vi "220121_xiang_calibration data analysis.vi"() -> ()   [LabVIEW 2020]
uses:
  OldDAQtask/CylinderCalibration/XYZE_power_spectra.ctl
  OldDAQtask/CylinderCalibration/single_power_spectrum.ctl
  OldDAQtask/CylinderCalibration/XYZ scan data.ctl
  OldDAQtask/CylinderCalibration/fast winding result.ctl
  <vilib>/Analysis/baseanly.llb/Mean (DBL).vi
  <vilib>/Utility/file.llb/Write To Spreadsheet File (DBL).vi
  Initialization/FileManagement/FileManagement.lvlib
  OldDAQtask/HeightFinder/HeightFinder.lvlib
  <vilib>/Analysis/NI_AALPro.lvlib
  <vilib>/Analysis/NI_AALBase.lvlib
  OldDAQtask/CylinderCalibration/CylinderCalibration.lvlib
panel:
  out "Array 2":dbl[][](array[numeric])
  out "Array":dbl[][](array[numeric])
  out "error out":errorcluster
  out "pb1":dbl(slide)=1.0 scale=0.0..1.0
  in  "kT_pNnm":dbl=4.09
  in  "stop":bool
  in  "cylinder list":i32[](listbox)
  in  "root path":path=path "Y:/Setup4/Xiaomeng/220107_Xiaomeng_q30 calibration"
  in  "Tab Control":T1(tab)=enum."averaged result"
  out "ellipticity vs angle":cluster{dbl[], dbl[]}[](graph)
  out "max ellipticity vs power":cluster{dbl[], dbl[]}[](graph)
  out "x variance vs angle":cluster{dbl[], dbl[]}[](graph)
  out "y variance vs angle":cluster{dbl[], dbl[]}[](graph)
  out "z variance vs angle":cluster{dbl[], dbl[]}[](graph)
  out "ellipticity fitting":cluster{dbl[], dbl[]}[](graph)
  out "z signal fitting":cluster{dbl[], dbl[]}[](graph)
  out "x signal fitting":cluster{dbl[], dbl[]}[](graph)
  out "y signal fitting":cluster{dbl[], dbl[]}[](graph)
  out "var ellipticity vs power":cluster{dbl[], dbl[]}[](graph)
  out "var x signal vs power":cluster{dbl[], dbl[]}[](graph)
  out "var y signal vs power":cluster{dbl[], dbl[]}[](graph)
  out "var z signal vs power":cluster{dbl[], dbl[]}[](graph)
  out "x DoG":cluster{dbl[], dbl[]}[](graph)
  out "y DoG":cluster{dbl[], dbl[]}[](graph)
  out "z DoG":cluster{dbl[], dbl[]}[](graph)
  out "Height finder data":cluster{dbl[], "Best Polynomial Fit":dbl[]}[](graph)
  out "original calibration file":string="[Trap and cylinder calibration]\nKz, pN/nm/W=0.349554\nKx, pN/nm/W=0.376339\nKy, pN/nm/W=0.248999\nSz, 1/nm=0.000578\nSx, 1/nm=0.000761\nSy, 1/nm=0.000667\nKang, pNnm/rad/W=17149.300335\nMax ellipticity, 1=0.032157\nFocal shift=0.790000\nZsignalHeightDependence, 1/nm=0\n[Piezo AO calibration and settings]\nVx/Px(V/nm)=0.000667\nVy/Py(V/nm)=0.000667\nVz/Pz(V/nm)=0.002000\nMax Px (nm)=30000.000000\nMax Py (nm)=30000.000000\nMax Pz (nm)=10000.000000\nMin Px (nm)=0.000000\nMin Py (nm)=0.000000\nMin Pz (nm)=0.000000\nVx0 (V)=-10.000000\nVy0 (V)=-10.000000\nVz0 (V)=-10.000000\nAI2p=1.101000E+4\\095.746000E+3\\093.323000E+0\\0D\\0A1.016000E+4\\095.766000E+3\\093.739000E+0\\0D\\0A6.154000E+3\\095.319000E+3\\091.621000E+1\\0D\\0A\n[matrix Mp2s (3X3)]\na11=1.000000\na12=0.000000\na13=0.000000\na21=0.000000\na22=1.000000\na23=0.000000\na31=0.000000\na32=0.000000\na33=1.000000\n[DAQ settings]\nAIBufferSize=100000\nDAQ ScanRate=10000\nPoints to average=20\nSamping rate=500\n[PS detector signal to laser power (W) conversion matrix (2X2)]\na11=0.0152532\na12=-0.00000458129\na21=-0.0000113255\na22=0.0139626\n[Z bead vs Z signal polynomial coefficients (nm)]\na0=0.000000\na1=1773.000000\na2=0.000000\na3=0.000000\na4=0.000000\na5=0.000000\n[Z bead look up table]\n(Z signal, Z bead)=-1.000000E+2\\09-4.925198E+2\\0D\\0A-2.068564E-1\\09-4.740681E+2\\0D\\0A-2.031962E-1\\09-4.583933E+2\\0D\\0A-1.995359E-1\\09-4.445056E+2\\0D\\0A-1.958757E-1\\09-4.317229E+2\\0D\\0A-1.922155E-1\\09-4.195962E+2\\0D\\0A-1.885553E-1\\09-4.078497E+2\\0D\\0A-1.848951E-1\\09-3.963318E+2\\0D\\0A-1.812349E-1\\09-3.849767E+2\\0D\\0A-1.775747E-1\\09-3.737744E+2\\0D\\0A-1.739145E-1\\09-3.627475E+2\\0D\\0A-1.702543E-1\\09-3.519346E+2\\0D\\0A-1.665941E-1\\09-3.413777E+2\\0D\\0A-1.629339E-1\\09-3.311145E+2\\0D\\0A-1.592737E-1\\09-3.211728E+2\\0D\\0A-1.556135E-1\\09-3.115682E+2\\0D\\0A-1.519532E-1\\09-3.023034E+2\\0D\\0A-1.482930E-1\\09-2.933685E+2\\0D\\0A-1.446328E-1\\09-2.847427E+2\\0D\\0A-1.409726E-1\\09-2.763963E+2\\0D\\0A-1.373124E-1\\09-2.682934E+2\\0D\\0A-1.336522E-1\\09-2.603938E+2\\0D\\0A-1.299920E-1\\09-2.526561E+2\\0D\\0A-1.263318E-1\\09-2.450395E+2\\0D\\0A-1.226716E-1\\09-2.375059E+2\\0D\\0A-1.190114E-1\\09-2.300210E+2\\0D\\0A-1.153512E-1\\09-2.225562E+2\\0D\\0A-1.116910E-1\\09-2.150888E+2\\0D\\0A-1.080307E-1\\09-2.076026E+2\\0D\\0A-1.043705E-1\\09-2.000879E+2\\0D\\0A-1.007103E-1\\09-1.925414E+2\\0D\\0A-9.705012E-2\\09-1.849654E+2\\0D\\0A-9.338991E-2\\09-1.773671E+2\\0D\\0A-8.972970E-2\\09-1.697580E+2\\0D\\0A-8.606949E-2\\09-1.621523E+2\\0D\\0A-8.240929E-2\\09-1.545665E+2\\0D\\0A-7.874908E-2\\09-1.470176E+2\\0D\\0A-7.508887E-2\\09-1.395227E+2\\0D\\0A-7.142866E-2\\09-1.320976E+2\\0D\\0A-6.776845E-2\\09-1.247560E+2\\0D\\0A-6.410824E-2\\09-1.175090E+2\\0D\\0A-6.044804E-2\\09-1.103642E+2\\0D\\0A-5.678783E-2\\09-1.033255E+2\\0D\\0A-5.312762E-2\\09-9.639297E+1\\0D\\0A-4.946741E-2\\09-8.956269E+1\\0D\\0A-4.580720E-2\\09-8.282687E+1\\0D\\0A-4.214700E-2\\09-7.617425E+1\\0D\\0A-3.848679E-2\\09-6.959053E+1\\0D\\0A-3.482658E-2\\09-6.305893E+1\\0D\\0A-3.116637E-2\\09-5.656087E+1\\0D\\0A-2.750616E-2\\09-5.007675E+1\\0D\\0A-2.384595E-2\\09-4.358670E+1\\0D\\0A-2.018575E-2\\09-3.707141E+1\\0D\\0A-1.652554E-2\\09-3.051286E+1\\0D\\0A-1.286533E-2\\09-2.389508E+1\\0D\\0A-9.205121E-3\\09-1.720474E+1\\0D\\0A-5.544913E-3\\09-1.043171E+1\\0D\\0A-1.884705E-3\\09-3.569408E+0\\0D\\0A1.775503E-3\\093.384973E+0\\0D\\0A5.435712E-3\\091.043038E+1\\0D\\0A9.095920E-3\\091.756204E+1\\0D\\0A1.275613E-2\\092.477176E+1\\0D\\0A1.641634E-2\\093.204839E+1\\0D\\0A2.007654E-2\\093.937846E+1\\0D\\0A2.373675E-2\\094.674700E+1\\0D\\0A2.739696E-2\\095.413840E+1\\0D\\0A3.105717E-2\\096.153747E+1\\0D\\0A3.471738E-2\\096.893042E+1\\0D\\0A3.837759E-2\\097.630600E+1\\0D\\0A4.203779E-2\\098.365648E+1\\0D\\0A4.569800E-2\\099.097859E+1\\0D\\0A4.935821E-2\\099.827434E+1\\0D\\0A5.301842E-2\\091.055516E+2\\0D\\0A5.667863E-2\\091.128245E+2\\0D\\0A6.033884E-2\\091.201134E+2\\0D\\0A6.399904E-2\\091.274448E+2\\0D\\0A6.765925E-2\\091.348504E+2\\0D\\0A7.131946E-2\\091.423665E+2\\0D\\0A7.497967E-2\\091.500322E+2\\0D\\0A7.863988E-2\\091.578880E+2\\0D\\0A8.230008E-2\\091.659733E+2\\0D\\0A8.596029E-2\\091.743245E+2\\0D\\0A8.962050E-2\\091.829723E+2\\0D\\0A9.328071E-2\\091.919395E+2\\0D\\0A9.694092E-2\\092.012384E+2\\0D\\0A1.006011E-1\\092.108698E+2\\0D\\0A1.042613E-1\\092.208213E+2\\0D\\0A1.079215E-1\\092.310681E+2\\0D\\0A1.115818E-1\\092.415750E+2\\0D\\0A1.152420E-1\\092.523003E+2\\0D\\0A1.189022E-1\\092.632031E+2\\0D\\0A1.225624E-1\\092.742540E+2\\0D\\0A1.262226E-1\\092.854502E+2\\0D\\0A1.298828E-1\\092.968364E+2\\0D\\0A1.335430E-1\\093.085323E+2\\0D\\0A1.372032E-1\\093.207678E+2\\0D\\0A1.408634E-1\\093.339281E+2\\0D\\0A1.445236E-1\\093.486096E+2\\0D\\0A1.481838E-1\\093.656889E+2\\0D\\0A1.000000E+2\\093.864067E+2\\0D\\0A\n[Comment from Q30 Calibration] 10 mM Tris-HCl, pH = 8; 40 mM MgCl2; 50 mM NaCl; 0.2 mg/mL beta-casein\n1/14/2021 11:33 AM"
  out "Updated calibration file":string
  out "Updated calibration file location":path
  out "SD of force sensitivity, pN/W":dbl=12.607172653733816
  out "SEM of force sensitivity, pN/W":dbl=3.151793163433454
  out "force sensitivity, pN/W":dbl=492.26794237481425
  out "SD of torque sensitivity, pNnm/W":dbl=244140.75454887396
  out "SEM of torque sensitivity, pNnm/W":dbl=61035.18863721849
  out "torque sensitivity, pNnm/W":dbl=308105.85527126427
  out "SD of z stiffness, pN/nm/W":dbl=0.006440898726546468
  out "SD of z sensitivity, 1/nm":dbl=5.569909992065383e-06
  out "SD of angular stifness, pNnm/rad/W":dbl=320.0752807876521
  out "SD of angular sensitivity, 1/rad":dbl=0.00035066082703313163
  out "z force sensitivity":T2(graph)={"final result"=[1.0, 2.0, 3.0, 4.0, 6.0, 7.0], "final result"=[498.4071904780335, 474.8213008025603, 504.1808261472068, 495.5040400134854, 478.2463154671384, 502.4479813404608]}
  out "Torque sensitivity":T2(graph)={"final result"=[1.0, 2.0, 3.0, 4.0, 6.0, 7.0], "final result"=[73.67021354183011, -8913.301705379306, 498179.1915137824, 417955.8385778271, 442478.0259262357, 498861.70710157783]}
  out "SEM of z stiffness, pN/nm/W":dbl=0.001610224681636617
  out "z stiffness, pN/nm/W":dbl=0.16169724642273595
  out "SEM of z sensitivity, 1/nm":dbl=1.3924774980163457e-06
  out "z sensitivity, 1/nm":dbl=0.00032838353115096313
  out "SEM of angular stifness, pNnm/rad/W":dbl=80.01882019691303
  out "angular stiffness, pNnm/rad/W":dbl=375.5197105345397
  out "SEM of angular sensitivity, 1/rad":dbl=8.766520675828291e-05
  out "angular sensitivity, 1/rad":dbl=0.0013622152574613259
  out "final result":dbl[][](array[numeric])=[[1.0, 2.0, 3.0, 4.0, 6.0, 7.0], [nan, nan, nan, nan, nan, nan], [0.13279234841776086, -13.36709953944761, 674.8537139952265, 372.11897404124767, 711.6919827860539, 507.68789957574], [0.0018025242772285583, 0.001499679914501309, 0.0013546405098627172, 0.0008903308428647679, 0.0016084233364951283, 0.001017692663815475], [73.67021354183011, -8913.301705379306, 498179.1915137824, 417955.8385778271, 442478.0259262357, 498861.70710157783], [0.16579227343626485, 0.1513303954658166, 0.16883942461520451, 0.16284381884534085, 0.15689235695361436, 0.16448520922017446], [0.00033264422464942726, 0.00031871020784036524, 0.0003348787098974448, 0.00032864276715263306, 0.0003280576386675683, 0.00032736763869834043], [498.4071904780335, 474.8213008025603, 504.1808261472068, 495.5040400134854, 478.2463154671384, 502.4479813404608], [0.6695465077566299, 0.9654608095555708, 1.1766726492381052, 1.2199767576089258, 1.1806760501666687, 0.7481024842794938], [0.0006195077361526612, 0.0007552886971877524, 0.0008161495017131666, 0.0008342978728837841, 0.0008284250298047227, 0.0006508474644543304], [1080.771826861639, 1278.267254826366, 1441.7366509054655, 1462.279597324187, 1425.205670626561, 1149.428284101409], [0.7539490293969152, 0.9600841428867122, 1.1413404013712398, 1.013487614262731, 1.027256013548298, 0.8640080844160597], [0.0005940302228699274, 0.0006707172355041432, 0.0007217134695992056, 0.0007028215814044456, 0.000725406642994016, 0.0006430202724935601], [1269.2098825449907, 1431.4290614062822, 1581.4314813953365, 1442.0268828932126, 1416.1105684233055, 1343.6716093965963], [0.19148344824695612, 0.21192606642906414, 0.19576149623991493, 0.19479979524743082, 0.19336718080202564, 0.19576422973039367], [0.12166886063179862, 0.12359792221219097, 0.12170898606033095, 0.12101974277514069, 0.11972394587250185, 0.12216359051715364]]
  out "z sensitivity":T2(graph)={"final result"=[1.0, 2.0, 3.0, 4.0, 6.0, 7.0], "final result"=[0.00033264422464942726, 0.00031871020784036524, 0.0003348787098974448, 0.00032864276715263306, 0.0003280576386675683, 0.00032736763869834043]}
  out "Angular sensitivity":T2(graph)={"final result"=[1.0, 2.0, 3.0, 4.0, 6.0, 7.0], "final result"=[0.0018025242772285583, 0.001499679914501309, 0.0013546405098627172, 0.0008903308428647679, 0.0016084233364951283, 0.001017692663815475]}
  out "max z force, pN/W":dbl=97.02091670635467
  out "SEM of max z force, pN/W":dbl=0.7160625967795665
  out "SD of max z force, pN/W":dbl=2.864250387118266
  out "Maximum torque":T2(graph)={"final result"=[1.0, 2.0, 3.0, 4.0, 6.0, 7.0], "final result"=[0.06639617420888043, -6.683549769723805, 337.42685699761324, 186.05948702062383, 355.84599139302696, 253.84394978787]}
  out "Maximum z force":T2(graph)={"final result"=[1.0, 2.0, 3.0, 4.0, 6.0, 7.0], "final result"=[95.43672746381132, 100.62701053581804, 98.69919290205362, 96.52408553890173, 92.47714175083674, 98.36134204670653]}
  out "Angular stiffness":T2(graph)={"final result"=[1.0, 2.0, 3.0, 4.0, 6.0, 7.0], "final result"=[0.13279234841776086, -13.36709953944761, 674.8537139952265, 372.11897404124767, 711.6919827860539, 507.68789957574]}
  out "z stiffness":T2(graph)={"final result"=[1.0, 2.0, 3.0, 4.0, 6.0, 7.0], "final result"=[0.16579227343626485, 0.1513303954658166, 0.16883942461520451, 0.16284381884534085, 0.15689235695361436, 0.16448520922017446]}
  out "CV of max z force":dbl=0.029521988498493166
  out "CV of angular sensitivity":dbl=0.2574195415243226
  out "CV of angular stifness":dbl=0.8523528108072828
  out "CV of z sensitivity":dbl=0.016961599665315758
  out "CV of z stiffness":dbl=0.03983307612862866
  out "CV of torque sensitivity":dbl=0.7923924533466792
  out "CV of force sensitivity":dbl=0.02561038728809742
  out "mean":dbl[](array[numeric])=[3.8333333333333335, nan, 375.5197105345397, 0.0013622152574613259, 308105.85527126427, 0.16169724642273595, 0.00032838353115096313, 492.26794237481425, 0.9934058764342324, 0.0007507527170327362, 1306.2815474409379, 0.960020880980326, 0.0006762849041442163, 1413.9799143432874, 0.1971837027826309, 0.12164717467818613]
  out "SD":dbl[](array[numeric])=[2.3166067138525404, nan, 320.0752807876521, 0.00035066082703313163, 244140.75454887396, 0.006440898726546468, 5.569909992065383e-06, 12.607172653733816, 0.2390944431916935, 9.435719400130207e-05, 163.137245645585, 0.13560242786564763, 5.115518013146681e-05, 104.91643534205578, 0.007404277385621852, 0.0012781918494249795]
  out "x stiffness":T2(graph)={"final result"=[1.0, 2.0, 3.0, 4.0, 6.0, 7.0], "final result"=[0.6695465077566299, 0.9654608095555708, 1.1766726492381052, 1.2199767576089258, 1.1806760501666687, 0.7481024842794938]}
  out "Maximum x force":T2(graph)={"final result"=[1.0, 2.0, 3.0, 4.0, 6.0, 7.0], "final result"=[60.64063499615816, 58.68692620128618, 61.36333714143654, 59.96577146647502, 57.25753598671112, 61.38084944864651]}
  out "x sensitivity":T2(graph)={"final result"=[1.0, 2.0, 3.0, 4.0, 6.0, 7.0], "final result"=[0.0006195077361526612, 0.0007552886971877524, 0.0008161495017131666, 0.0008342978728837841, 0.0008284250298047227, 0.0006508474644543304]}
  out "x force sensitivity":T2(graph)={"final result"=[1.0, 2.0, 3.0, 4.0, 6.0, 7.0], "final result"=[1080.771826861639, 1278.267254826366, 1441.7366509054655, 1462.279597324187, 1425.205670626561, 1149.428284101409]}
  out "max x force, pN/W":dbl=59.882509206785585
  out "SD of max x force, pN/W":dbl=1.6333686233039957
  out "SEM of max x force, pN/W":dbl=0.4083421558259989
  out "CV of max x force":dbl=0.027276222137981327
  out "x stiffness, pN/nm/W":dbl=0.9934058764342324
  out "SEM of x stiffness, pN/nm/W":dbl=0.05977361079792338
  out "SD of x stiffness, pN/nm/W":dbl=0.2390944431916935
  out "CV of x stiffness":dbl=0.24068152692020295
  out "z sensitivity, 1/nm 2":dbl=0.0007507527170327362
  out "SEM of z sensitivity, 1/nm 2":dbl=2.358929850032552e-05
  out "SD of z sensitivity, 1/nm 2":dbl=9.435719400130207e-05
  out "CV of z sensitivity 2":dbl=0.1256834532337599
  out "Comment":string
  out "Name":string
  in  "fast winding results":T3[](array[typedef]) {"Laser power before obj[W]" format="%.4f"; "relative fluctuation (fluctuation/mean)" format="%#_6e"; "mean e amplitude" format="%#_6e"}
  in  "stifness results":T4[][](array[typedef]) {"result of y signal"."var" format="%.3e"; "result of y signal"."sigma^2" format="%.3e"; "result of x signal"."var" format="%.3e"; "result of x signal"."sigma^2" format="%.3e"; "result of z signal"."var" format="%.3e"; "result of z signal"."sigma^2" format="%.3e"; "result of ellipticity"."var" format="%.3e"; "result of ellipticity"."sigma^2" format="%.3e"; "general info"."Time/Date" format="%<%.3X, %x>T"}
  in  "XYZ scan result":T6 {"y_signal vs trap height slope around eq position, 1/nm" format="%#.6g"; "x_signal vs trap height slope around eq position, 1/nm" format="%#.6g"; "Zsig baseline" format="%#.6g"; "Xsig baseline" format="%#.6g"; "Ysig baseline" format="%#.6g"; "z_signal vs trap height slope around eq position, 1/nm" format="%#.6g"}
  out "distance between trap center and z DoG center":dbl[](array[numeric])
  out "only use slopes":dbl[][](array[numeric]) format="%_3e"
  out "intercepts that will be ignored":dbl[][](array[numeric]) format="%_3e"
  # "column name:\n\n0: Cylinder No.\n1: Good? (=1)\n2: K_theta\n3: S_theta\n4: K_e\n5: K_z\n6: S_z\n7: K_zsig\n8: K_x\n9: S_x\n10: K_xsig\n11: K_y\n12: S_y\n13: K_ysig\n14: Max z signal\n15: Max x signal"
  # "Rows:\n\n0: Cylinder No.\n1: \n2: K_theta\n3: S_theta\n4: K_e\n5: K_z\n6: S_z\n7: K_zsig\n8: K_x\n9: S_x\n10: K_xsig\n11: K_y\n12: S_y\n13: K_ysig\n14: Max z signal\n15: Max x signal"
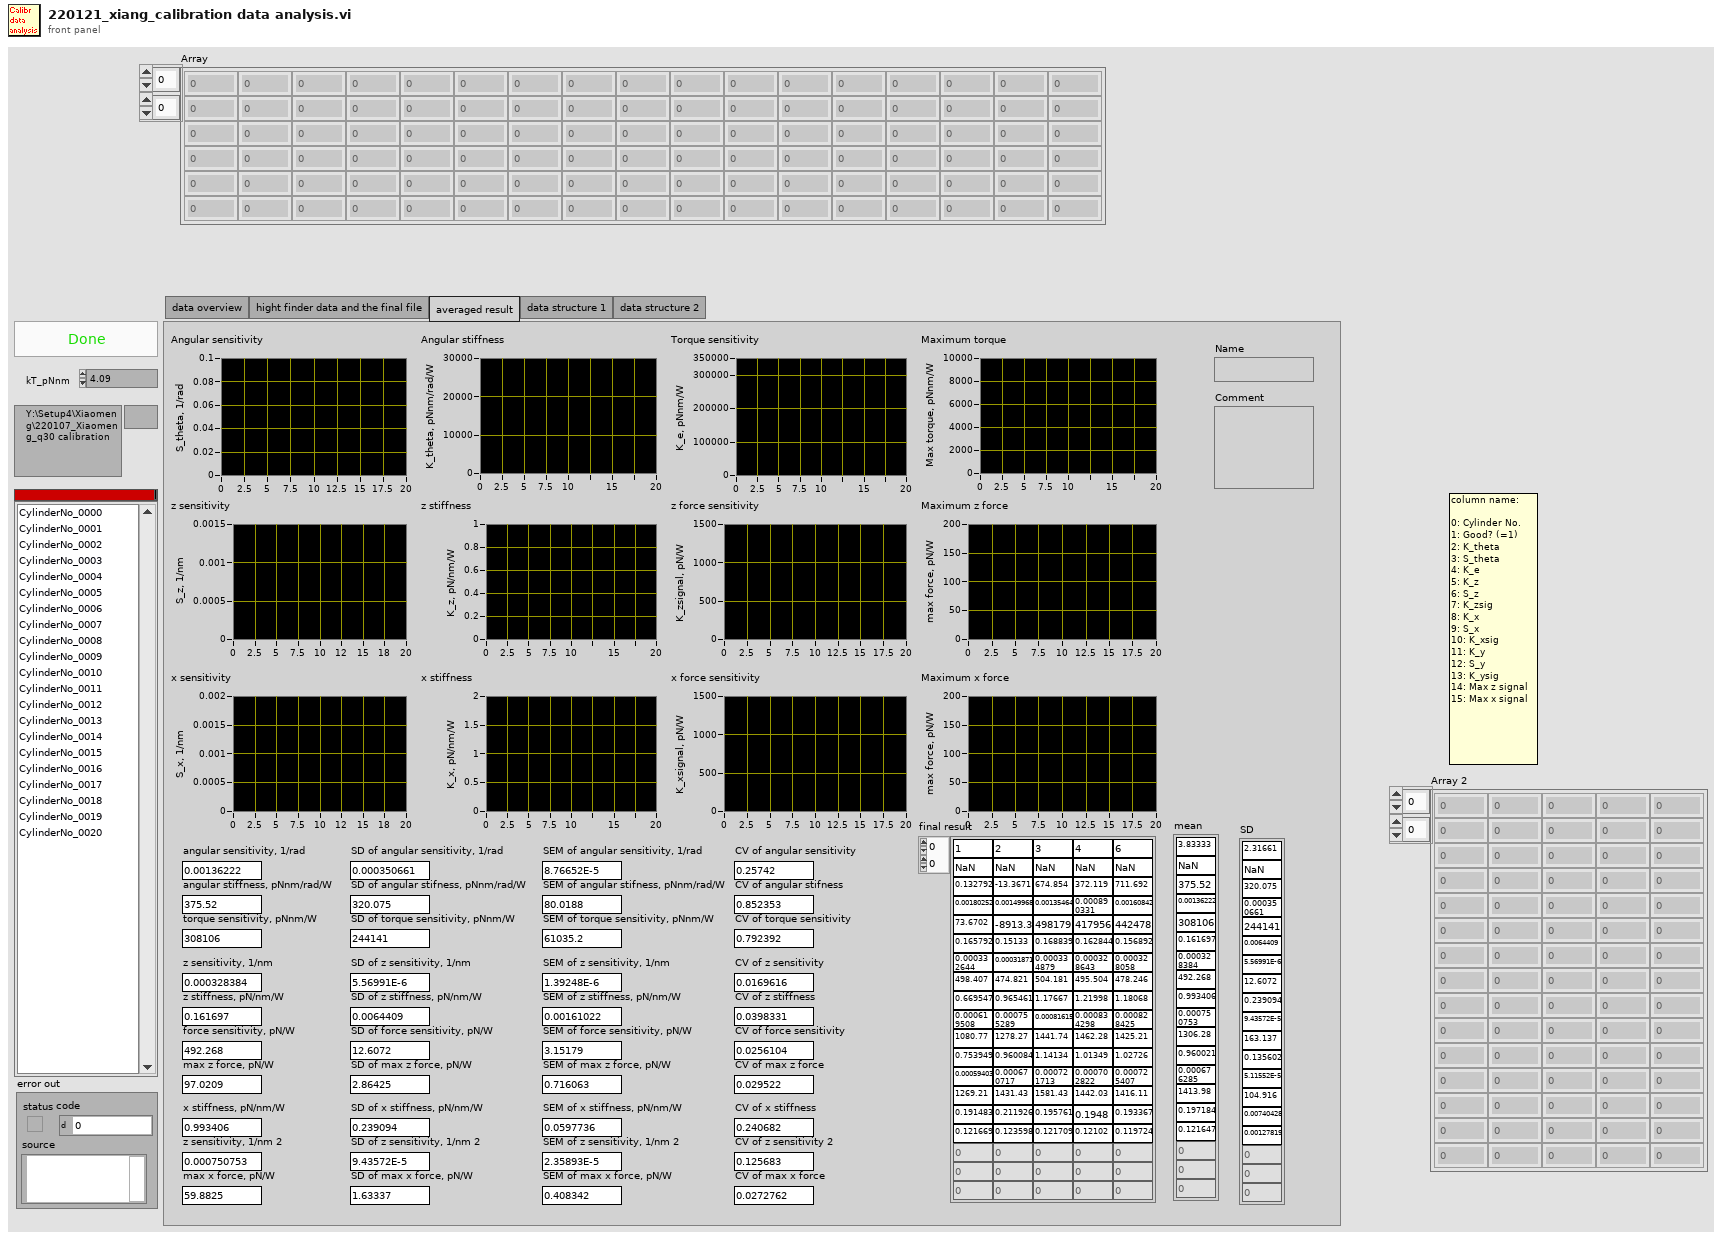
[diagram p1: front panel]
types:
  T1 = enum32{"data overview", "hight finder data and the final file", "averaged result", "data structure 1", "data structure 2"}
  T2 = cluster{"final result":dbl[], "final result":dbl[]}
  T3 = typedef "CylinderCalibration.lvlib/fast winding result.ctl" = cluster{"fast pol (current file)":dbl[], "fit fast pol fitting result":cluster{dbl[], "best nonlinear fit":dbl[]}[], "fit result: amplitude":dbl[], "mean e amplitude":dbl, "relative fluctuation (fluctuation/mean)":dbl, "Laser power before obj[W]":dbl}
  T4 = typedef "CylinderCalibration.lvlib/XYZE_power_spectra.ctl" = cluster{"general info":cluster{"Time/Date ":timestamp, "Laser power before obj[W]":dbl, "Cylinder height  [nm]":dbl, "Polarization angle (turn)":dbl}, "result of ellipticity":T5, "result of z signal":T5, "result of x signal":T5, "result of y signal":T5}
  T5 = typedef "CylinderCalibration.lvlib/single_power_spectrum.ctl" = cluster{"raw signal (linear drift removed)":dbl[], "signal distribution":cluster{"X Values":dbl[], "Best Gaussian Fit":dbl[]}[], "power":cluster{dbl[], "best nonlinear fit":dbl[]}[], "A and fc":dbl[], "cutoff %":dbl, "dt [s] ":dbl, "sigma^2":dbl, "var ":dbl}
  T6 = typedef "CylinderCalibration.lvlib/XYZ scan data.ctl" = cluster{"height finder result":cluster{"Y":dbl[], "Y":dbl[]}[], "Instrument Calibr.XYZsignal baseline.Zsignal0":dbl, "Z signal vs trap height, fitting":cluster{dbl[], "Best Polynomial Fit":dbl[]}[], "z_signal vs trap height slope around eq position, 1/nm":dbl, "Z signal Truncated data with redrawn polynomial":cluster{dbl[], "Best Polynomial Fit":dbl[]}[], "Z signal Residues":cluster{dbl[], dbl[]}, "Z center positon":dbl, "Zsig baseline":dbl, "X signal Truncated data with redrawn polynomial":cluster{dbl[], "Best Polynomial Fit":dbl[]}[], "X signal Residues":cluster{dbl[], dbl[]}, "X center positon":dbl, "Xsig baseline":dbl, "Y signal Truncated data with redrawn polynomial":cluster{dbl[], "Best Polynomial Fit":dbl[]}[], "Y signal Residues":cluster{dbl[], dbl[]}, "Y center positon":dbl, "Ysig baseline":dbl, "x_signal vs trap height slope around eq position, 1/nm":dbl, "y_signal vs trap height slope around eq position, 1/nm":dbl}
  T7 = enum32{"result overview", "XYZ sensitivity", "averaged result", "averaged result 2", "config.ini", "data format", "data format 2"}
  T8 = enum16{"deny read/write", "deny write-only", "deny none"}
  T9 = typedef "Initialization.lvlib/Param.ctl" = cluster{"TaskIDs":cluster{"DAQ tasks":cluster{"Px taskID":u32, "Py taskID":u32, "Pz taskID":u32, "AOM taskID":u32, "Clock taskID":u32, "AI taskID":u32}, "DVEHandle":refnum<file>}, "Manual Control":T10, "Piezo Calibr":cluster{"Px2Vx(AO)":dbl, "Py2Vy(AO)":dbl, "Pz2Vz(AO)":dbl, "Min Px":dbl, "Min Py":dbl, "Min Pz":dbl, "Max Px":dbl, "Max Py":dbl, "Max Pz":dbl, "Vx0 (V)":dbl, "Vy0 (V)":dbl, "Vz0 (V)":dbl}, "Instrument Calibr":cluster{"Angular compensation coeffs":dbl[][], "TetherCenter":cluster{"TrapX_AO 0 [nm]":dbl, "TrapY_AO 0 [nm]":dbl, "TrapZ_AO 0 [nm]":dbl}, "XYZsignal baseline":cluster{"Xsignal0":dbl, "Ysignal0":dbl, "Zsignal0":dbl, "Zsig slope":dbl, "Z bead0":dbl}, "S and P to Vs0":cluster{"Vs0/P":dbl, "Vs0/S":dbl}, "Psi":dbl, "ePS:eRL drift correlation":cluster{"Interc P":dbl, "Slope P":dbl, "Interc S":dbl, "Slope S":dbl}, "Current piezo volt AO":cluster{"Vpx_AO [V]":dbl, "Vpy_AO [V]":dbl, "Vpz_AO [V]":dbl}}, "Cylinder Calibr":T12, "DAQParams":cluster{"Buffer size":dbl, "Scanning rate":dbl, "Average":dbl, "Sampling rate":dbl, "set dt":dbl}, "DAQ channel offsets":T13, "Z bead polynomial coeffs":dbl[], "Skip button ref":refnum<vi>, "z bead lookup table":cluster{"z signal":dbl[], "z bead":dbl[]}, "SP->power Matrix":T14, "Ms2p":T14, "Mp2s":T14, "Polynomial coeff V_px,y,z 2 position (nm)":dbl[][]}
  T10 = typedef "Initialization.lvlib/ManualCtrl.ctl" = cluster{"Rotation Control":T11, "X piezo\n [nm]":dbl, "Y peizo\n [nm]":dbl, "trap height\n [nm]":dbl, "AOM0 \nPower":dbl}
  T11 = typedef "Initialization.lvlib/DVESetting.ctl" = cluster{"Phase":dbl, "A amp (0-120)":dbl, "B amp (0-120)":dbl, "mean freq  [MHz]\ndefault 39.99":dbl, "freq difference [Hz]":dbl, "Enable A":bool, "Enable B":bool}
  T12 = typedef "Initialization.lvlib/CylinderCalibrNew.ctl" = cluster{"ZStiff":dbl, "Zsens":dbl, "AngStiff":dbl, "XStiff":dbl, "Xsens":dbl, "MaxEllip":dbl, "YStiff":dbl, "Ysens":dbl, "FocalShift":dbl, "Sfz":dbl, "1/Sz":dbl, "Stau":dbl, "Sfx":dbl, "1/Sx":dbl, "1/Sang":dbl, "Sfy":dbl, "1/Sy":dbl, "1/focal":dbl, "ZsignalHeightDependence (1/nm)":dbl}
  T13 = typedef "SignalConverson.lvlib/DAQChannelOffsets.ctl" = cluster{"A0 [V]":dbl, "D0 [V]":dbl, "P0  [V]":dbl, "S0 [V]":dbl, "L0 [V]":dbl, "R0 [V]":dbl, "Vpx0 [V]":dbl, "Vpy0 [V]":dbl, "Vpz0 [V]":dbl, "Vsum0 [V]":dbl, "Vpx_AO0 [V]":dbl, "Vpy_AO0 [V]":dbl, "Vpz_AO0 [V]":dbl}
  T14 = typedef "NI_Matrix.lvlib/RealMatrix.ctl" = dbl[][]
  T15 = cluster{"Time/Date ":timestamp, "Laser power before obj[W]":dbl, "Cylinder height  [nm]":dbl, "Polarization angle (turn)":dbl}
  T16 = cluster{"general info":cluster{"Time/Date ":timestamp, "Laser power before obj[W]":dbl, "Cylinder height  [nm]":dbl, "Polarization angle (turn)":dbl}, "A and fc":dbl[], "var ":dbl, "A and fc":dbl[], "var ":dbl, "A and fc":dbl[], "var ":dbl, "A and fc":dbl[], "var ":dbl}
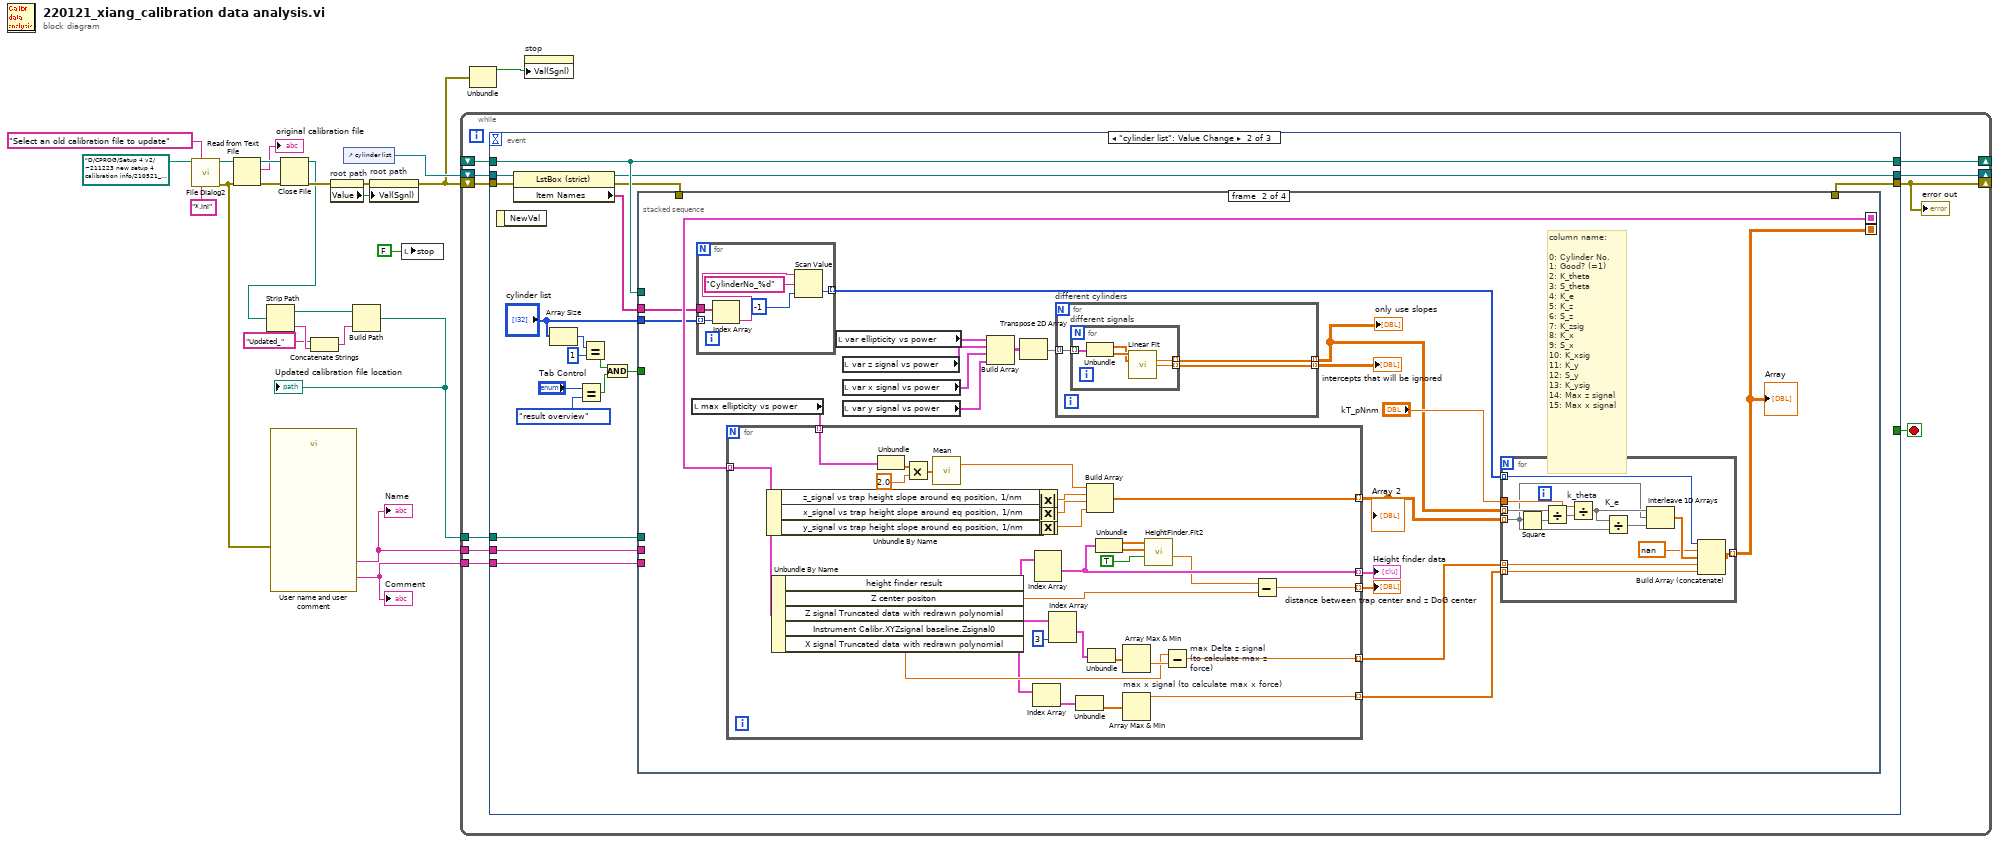
[diagram p0: block diagram]
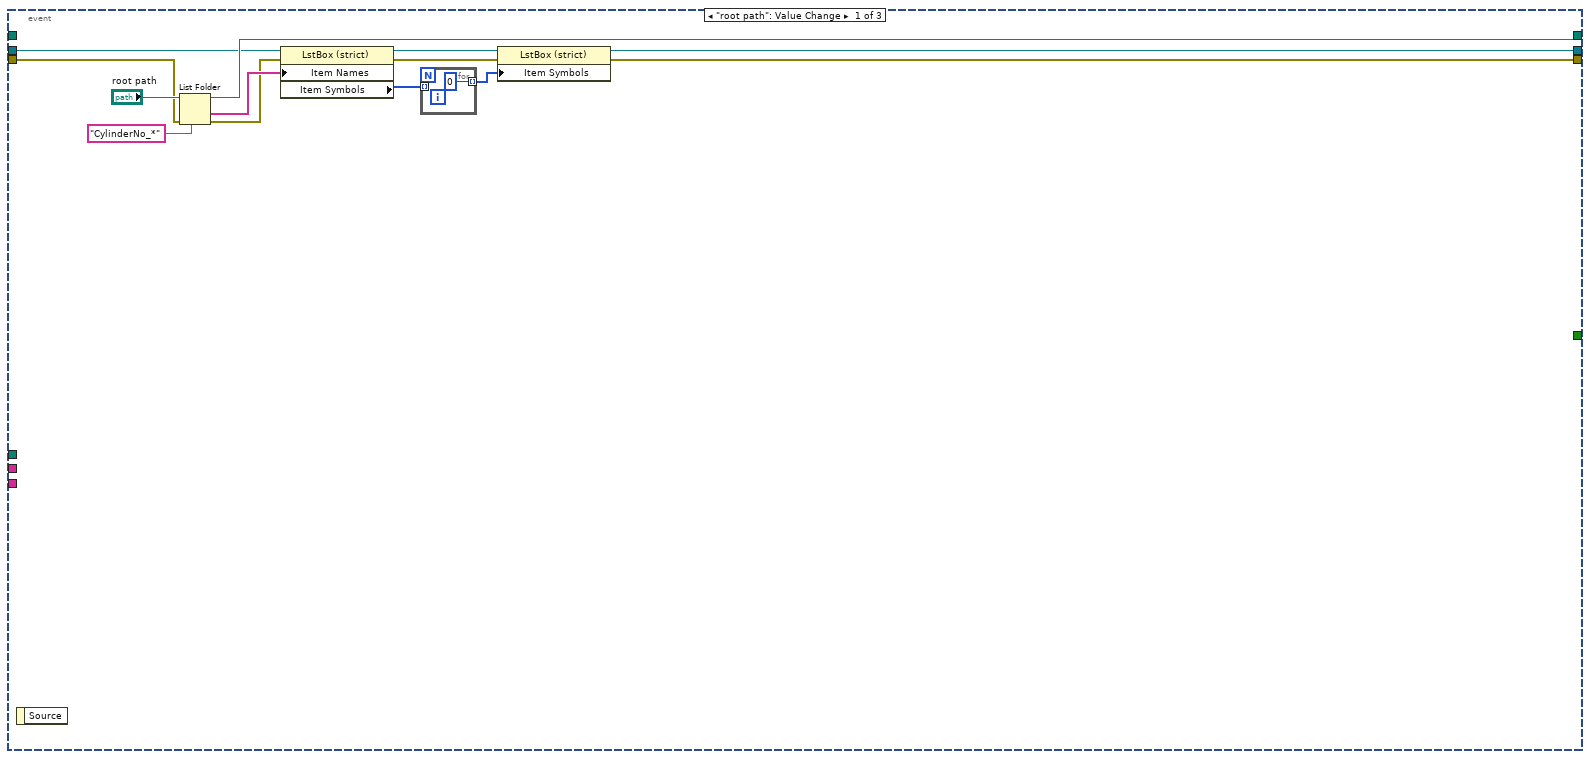
[diagram p2: hidden frame]
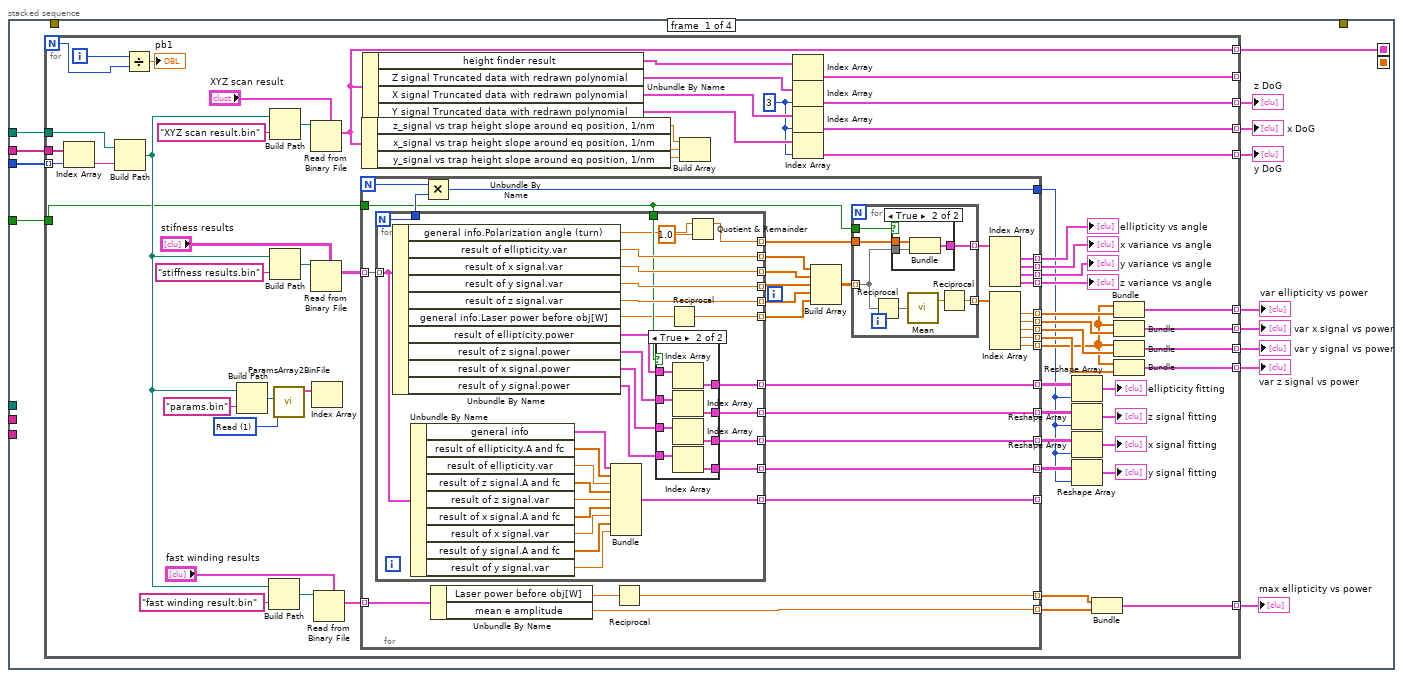
[diagram p3: hidden frame]
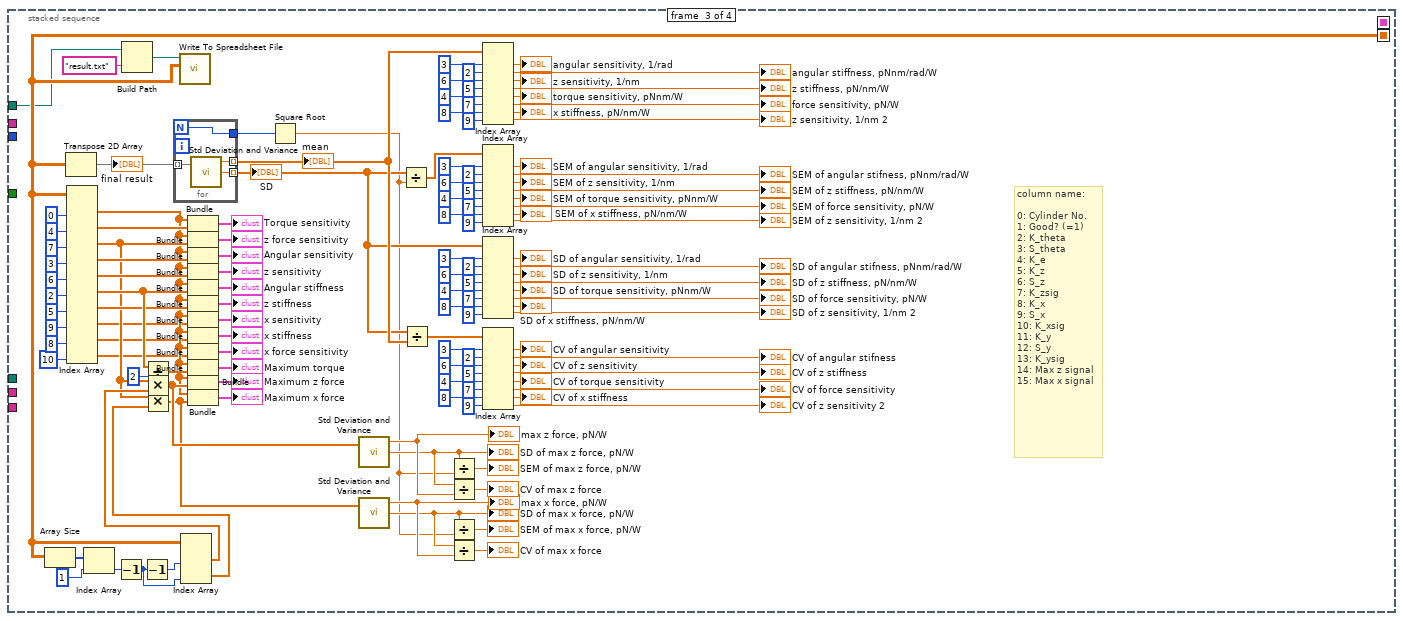
[diagram p6: hidden frame]
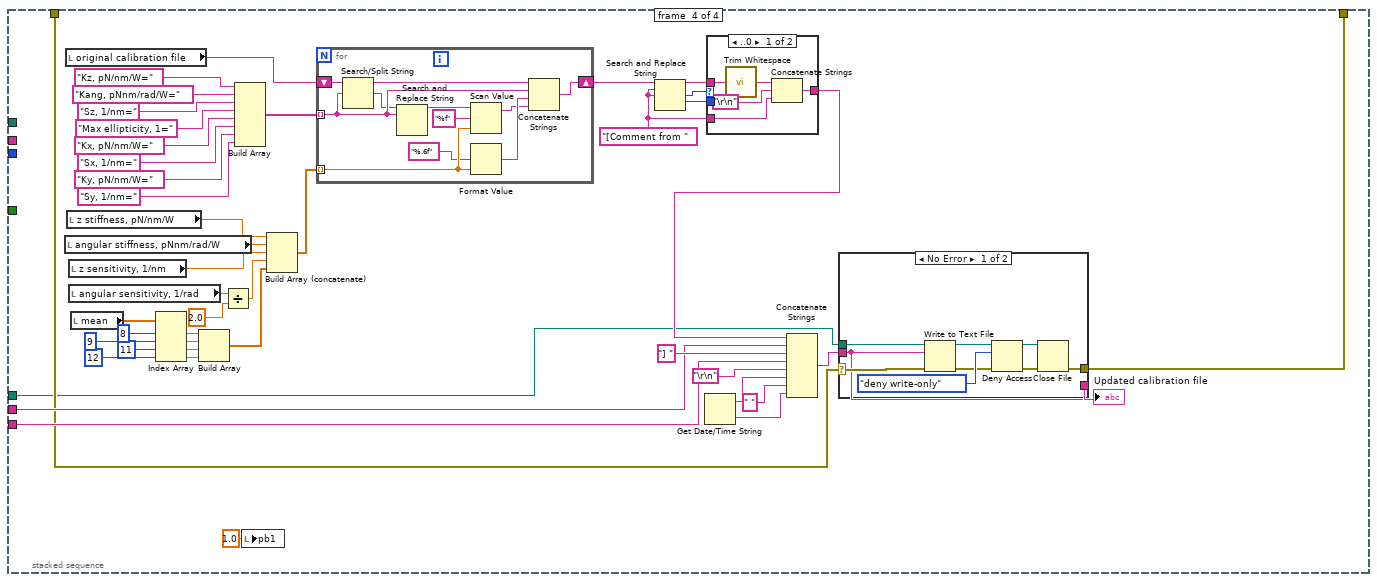
[diagram p7: hidden frame]
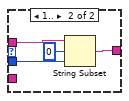
[diagram p8: hidden frame]
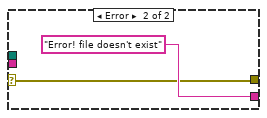
[diagram p9: hidden frame]
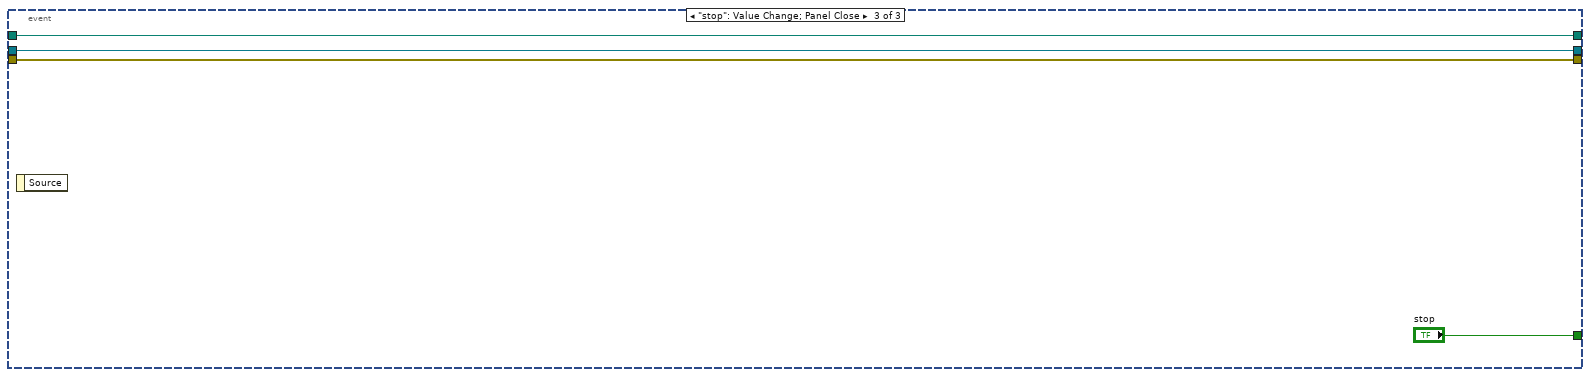
[diagram p10: hidden frame]
diagram:
  n1 = call "File Dialog2"("start path"=path "D:/CPROG/Setup 4 v2/~211223 new setup 4 calibration info/210521_PSbead Config_Xiang (xiang modified 220119).ini", "prompt"="Select an old calibration file to update", "pattern (all files)"="*.ini") -> ("selected path"=w17:path, "error out"=w5:errorcluster)  [unwired: 9 in, 2 out]
  n2 = Read from Text File(file (use dialog)=w17, error in=w5) -> (refnum out=w19:refnum<file>, text=→"original calibration file":string, error out=w16:errorcluster)  [unwired: 2 in, 1 out]
  n3 = call "User name and user comment"("error in (no error)"=w5) -> ("Comment"=w1:string, "Name"=w2:string)  [unwired: 15 in, 2 out]
  "Name" <- w2
  "Comment" <- w1
  n4 = Close File(refnum=w19, error in=w16) -> (path=w3:path, error out=w11:errorcluster)
  n5 = Strip Path(path=w3) -> (stripped path=w7:path, name=w9:string)
  n6 = Concatenate Strings("Updated_" ("name"), w9) -> (w10:string)
  n7 = property on="root path" class="Path"(error in=w11) -> (error out=w23:errorcluster, "Value"=w22:path)  [unwired: 1 in, 1 out]
  n8 = control-ref of="cylinder list"() -> (w21:refnum<vi>)
  n9 = Build Path(base path=w7, name or relative path=w10) -> (appended path=w6:path)
  "Updated calibration file location" <- w6
  n10 = property on="root path" class="Path"(error in=w23, "Val(Sgnl)"=w22) -> (error out=w14:errorcluster)  [unwired: 1 in, 1 out]
  n11 = local write "stop"(FALSE ("stop")) -> ()
  n12 = while {
    shift-right: [w28] -> _
    shift-left: _ -> [w31]
    shift-right: [w29] -> _
    shift-left: w21 -> [w33]
    shift-right: [w24] -> _
    shift-left: w14 -> [w32]
    tunnel: w2 -> [w27]
    tunnel: w1 -> [w26]
    tunnel: w6 -> [w25]
    stop <- w30 stop-if-true
    n13 = event shown="[1] \"cylinder list\": Value Change" {
      selector: _ -> [_ _ _]
      dyn-events: _ -> [_ _ _]
      timeout: _ -> [_ _ _]
      tunnel: w33 -> [w36 w65 w508]
      tunnel: w32 -> [w35 w54 w507]
      tunnel: w31 -> [_ w63 w509]
      tunnel: [_ _ "stop"] -> w30
      tunnel: [w40 w62 w508] -> w29
      tunnel: [w38 w49 w507] -> w24
      tunnel: [w43 w63 w509] -> w28
      tunnel: w27 -> [_ w51 _]
      tunnel: w26 -> [_ w50 _]
      tunnel: w25 -> [_ w48 _]
      event "root path": Value Change {
        n14 = event-data() -> ()  [unwired: 1 in, 1 out]
        n15 = List Folder(path="root path", pattern="CylinderNo_*", error in=w35) -> (path out=w43:path, folder names=w46:string[], error out=w34:errorcluster)  [unwired: 1 in, 1 out]
        n16 = property class="LstBox (strict)"(reference=w36, error in=w34, "Item Names"=w46) -> (reference out=w41:refnum<vi>, error out=w39:errorcluster, "Item Symbols"=w37:i32[])
        n17 = for {
          tunnel: [0] -> w42 mode=indexing
          tunnel: w37 -> [_] mode=indexing
        }
        n18 = property class="LstBox (strict)"(reference=w41, error in=w39, "Item Symbols"=w42) -> (reference out=w40:refnum<vi>, error out=w38:errorcluster)
      }
      event "cylinder list": Value Change {
        n19 = event-data() -> ()  [unwired: 1 in, 1 out]
        n20 = property class="LstBox (strict)"(reference=w65, error in=w54) -> (reference out=w62:refnum<vi>, error out=w52:errorcluster, "Item Names"=w64:string[])
        n21 = Array Size(array="cylinder list") -> (size(s)=w61:i32)
        n22 = Equal?(x="Tab Control", y=T7."result overview" ("Tab Control")) -> (x = y?=w57:bool)
        n23 = Equal?(x=w61, y=1) -> (x = y?=w56:bool)
        n24 = And(x=w56, y=w57) -> (x .and. y?=w55:bool)
        n25 = stacked-sequence {
          seq-local: [w66 _ _ _] -> [_ w231 _ _]
          seq-local: [_ w227 _ _] -> [_ _ w340 _]
          tunnel: w64 -> [w78 w230 _ _]
          tunnel: w63 -> [w77 _ w339 _]
          tunnel: "cylinder list" -> [w76 w229 _ _]
          tunnel: w55 -> [w75 _ _ _]
          tunnel: w52 -> [_ _ _ w432]
          tunnel: w51 -> [_ _ _ w435]
          tunnel: w50 -> [_ _ _ w434]
          tunnel: [_ _ _ w433] -> w49
          tunnel: w48 -> [_ _ _ w431]
          frame #0 {
            n26 = for {
              N -> [w82]
              tunnel: w78 -> [w140]
              tunnel: w77 -> [w128]
              tunnel: w76 -> [w124] mode=indexing
              tunnel: [w111] -> w73 mode=indexing
              tunnel: [w110] -> w72 mode=indexing
              tunnel: [w109] -> w71 mode=indexing
              tunnel: [w108] -> w70 mode=indexing
              tunnel: w75 -> [w102]
              tunnel: [w103] -> w74 mode=indexing
              tunnel: [w93] -> _ mode=indexing
              tunnel: [w92] -> w69 mode=indexing
              tunnel: [w91] -> w68 mode=indexing
              tunnel: [w90] -> w67 mode=indexing
              tunnel: [w81] -> w66 mode=indexing
              i -> [w79]
              w80 = 3 ("index")
              w129 = 1 items=["Write", "Read"] ("write (0) or read (1)")
              n27 = Index Array(array=w140, index=w124) -> (element=w86:string)
              n28 = Build Path(base path=w128, name or relative path=w86) -> (appended path=w139:path)
              n29 = Divide(x=w79, y=w82) -> (x/y=→"pb1":dbl)
              n30 = Build Path(base path=w139, name or relative path="params.bin") -> (appended path=w131:path)
              n31 = Build Path(base path=w139, name or relative path="fast winding result.bin") -> (appended path=w137:path)
              n32 = Build Path(base path=w139, name or relative path="XYZ scan result.bin") -> (appended path=w136:path)
              n33 = Build Path(base path=w139, name or relative path="stiffness results.bin") -> (appended path=w138:path)
              n34 = call "ParamsArray2BinFile.vi"("write (0) or read (1)"=w129, "file path in"=w131) -> ("Array of Params out"=w130:T9[])  [unwired: 6 in, 3 out]
              n35 = Read from Binary File(5:"XYZ scan result", 11:w136) -> (2:w81:T6)  [unwired: 4 in, 3 out]
              n36 = Read from Binary File(5:"stifness results", 11:w138) -> (2:w126:T4[][])  [unwired: 4 in, 3 out]
              n37 = Index Array(array=w130) -> ()  [unwired: 1 in, 1 out]
              n38 = Read from Binary File(5:"fast winding results", 11:w137) -> (2:w125:T3[])  [unwired: 4 in, 3 out]
              n39 = for {
                N -> [w151]
                tunnel: w126 -> [w172] mode=indexing
                tunnel: w125 -> [w171] mode=indexing
                tunnel: [w162] -> w120 mode=indexing
                tunnel: [w161] -> w119 mode=indexing
                tunnel: [w160] -> w118 mode=indexing
                tunnel: [w159] -> w117 mode=indexing
                tunnel: [w157] -> w112 mode=indexing
                tunnel: [w156] -> w113 mode=indexing
                tunnel: [w155] -> w114 mode=indexing
                tunnel: [w154] -> w115 mode=indexing
                tunnel: [w153] -> w116 mode=indexing
                tunnel: [w150] -> w101
                tunnel: [w149] -> w107 mode=indexing
                tunnel: [w148] -> w106 mode=indexing
                tunnel: [w147] -> w105 mode=indexing
                tunnel: [w146] -> w104 mode=indexing
                tunnel: [w143] -> w85 mode=indexing
                tunnel: [w141] -> w84 mode=indexing
                tunnel: w102 -> [w145]
                tunnel: [w142] -> _ mode=indexing
                n40 = for {
                  N -> [w200]
                  tunnel: w172 -> [w184] mode=indexing
                  tunnel: [w212] -> w166 mode=indexing
                  tunnel: [w211] -> w167 mode=indexing
                  tunnel: [w210] -> w168 mode=indexing
                  tunnel: [w209] -> w170 mode=indexing
                  tunnel: [w197] -> w164 mode=indexing
                  tunnel: [w194] -> w169 mode=indexing
                  tunnel: [w204] -> w146 mode=indexing
                  tunnel: [w203] -> w147 mode=indexing
                  tunnel: [w202] -> w148 mode=indexing
                  tunnel: [w201] -> w149 mode=indexing
                  tunnel: [w200] -> w152
                  tunnel: w145 -> [w199]
                  tunnel: [w183] -> w142 mode=indexing
                  n41 = Unbundle By Name(w184) -> ("general info.Polarization angle (turn)"=w196:dbl, "result of ellipticity.var"=w212:dbl, "result of x signal.var"=w211:dbl, "result of y signal.var"=w210:dbl, "result of z signal.var"=w209:dbl, "general info.Laser power before obj[W]"=w198:dbl, "result of ellipticity.power"=w208:cluster{dbl[], "best nonlinear fit":dbl[]}[], "result of z signal.power"=w207:cluster{dbl[], "best nonlinear fit":dbl[]}[], "result of x signal.power"=w206:cluster{dbl[], "best nonlinear fit":dbl[]}[], "result of y signal.power"=w205:cluster{dbl[], "best nonlinear fit":dbl[]}[])
                  n42 = Unbundle By Name(w184) -> ("general info"=w185:T15, "result of ellipticity.A and fc"=w186:dbl[], "result of ellipticity.var"=w187:dbl, "result of z signal.A and fc"=w188:dbl[], "result of z signal.var"=w189:dbl, "result of x signal.A and fc"=w190:dbl[], "result of x signal.var"=w191:dbl, "result of y signal.A and fc"=w192:dbl[], "result of y signal.var"=w193:dbl)
                  n43 = Bundle("general info"=w185, "A and fc"=w186, "var"=w187, "A and fc"=w188, "var"=w189, "A and fc"=w190, "var"=w191, "A and fc"=w192, "var"=w193) -> (w183:T16)  [unwired: 1 in]
                  n44 = case shown="True" w199 {
                    tunnel: w208 -> [_ w220]
                    tunnel: w207 -> [_ w219]
                    tunnel: w206 -> [_ w218]
                    tunnel: w205 -> [_ w217]
                    tunnel: [_ w216] -> w204
                    tunnel: [_ w215] -> w203
                    tunnel: [_ w214] -> w202
                    tunnel: [_ w213] -> w201
                    frame False {
                    }
                    frame True {
                      n45 = Index Array(array=w220) -> (element=w213:cluster{dbl[], "best nonlinear fit":dbl[]})  [unwired: 1 in]
                      n46 = Index Array(array=w219) -> (element=w214:cluster{dbl[], "best nonlinear fit":dbl[]})  [unwired: 1 in]
                      n47 = Index Array(array=w218) -> (element=w215:cluster{dbl[], "best nonlinear fit":dbl[]})  [unwired: 1 in]
                      n48 = Index Array(array=w217) -> (element=w216:cluster{dbl[], "best nonlinear fit":dbl[]})  [unwired: 1 in]
                    }
                  }
                  n49 = Reciprocal(x=w198) -> (1/x=w197:dbl)
                  n50 = Quotient & Remainder(x=w196, y=1.0) -> (x-y*floor(x/y)=w194:dbl)  [unwired: 1 out]
                }
                n51 = Multiply(x=w151, y=w152) -> (x*y=w150:i32)
                n52 = Unbundle By Name(w171) -> ("Laser power before obj[W]"=w144:dbl, "mean e amplitude"=w141:dbl)
                n53 = Reciprocal(x=w144) -> (1/x=w143:dbl)
                n54 = Build Array(w166, w167, w168, w170, w164) -> (w165:dbl[][])
                n55 = for {
                  tunnel: w165 -> [w176] mode=indexing
                  tunnel: [w173] -> w158 mode=indexing
                  tunnel: w169 -> [w179]
                  tunnel: [w178] -> w163 mode=indexing
                  tunnel: w145 -> [w177]
                  n56 = Reciprocal(x=w176) -> (1/x=w175:dbl[])
                  n57 = case shown="True" w177 {
                    tunnel: w176 -> [_ w182]
                    tunnel: w179 -> [_ w181]
                    tunnel: [_ w180] -> w178
                    frame False {
                    }
                    frame True {
                      n58 = Bundle(w181, w182) -> (w180:cluster{dbl[], dbl[]})  [unwired: 1 in]
                    }
                  }
                  n59 = call-poly <vilib>:"Mean.vi"("X"=w175) -> ("mean"=w174:dbl)  [unwired: 1 out]
                  n60 = Reciprocal(x=w174) -> (1/x=w173:dbl)
                }
                n61 = Index Array(array=w163) -> (element #1=w162:cluster{dbl[], dbl[]}, element #2=w161:cluster{dbl[], dbl[]}, element #3=w160:cluster{dbl[], dbl[]}, element #4=w159:cluster{dbl[], dbl[]})  [unwired: 4 in]
                n62 = Index Array(array=w158) -> (element #1=w153:dbl, element #2=w154:dbl, element #3=w155:dbl, element #4=w156:dbl, element #5=w157:dbl)  [unwired: 5 in]
              }
              "ellipticity vs angle" <- w120
              "x variance vs angle" <- w119
              "y variance vs angle" <- w118
              "z variance vs angle" <- w117
              n63 = Unbundle By Name(w81) -> ("z_signal vs trap height slope around eq position, 1/nm"=w87:dbl, "x_signal vs trap height slope around eq position, 1/nm"=w88:dbl, "y_signal vs trap height slope around eq position, 1/nm"=w89:dbl)
              n64 = Unbundle By Name(w81) -> ("height finder result"=w127:cluster{"Y":dbl[], "Y":dbl[]}[], "Z signal Truncated data with redrawn polynomial"=w96:cluster{dbl[], "Best Polynomial Fit":dbl[]}[], "X signal Truncated data with redrawn polynomial"=w95:cluster{dbl[], "Best Polynomial Fit":dbl[]}[], "Y signal Truncated data with redrawn polynomial"=w94:cluster{dbl[], "Best Polynomial Fit":dbl[]}[])
              n65 = Build Array(w87, w88, w89) -> ()  [unwired: 1 out]
              n66 = Index Array(array=w127) -> (element=w93:cluster{"Y":dbl[], "Y":dbl[]})  [unwired: 1 in]
              n67 = Index Array(array=w96, index=w80) -> (element=w92:cluster{dbl[], "Best Polynomial Fit":dbl[]})
              n68 = Index Array(array=w95, index=w80) -> (element=w91:cluster{dbl[], "Best Polynomial Fit":dbl[]})
              n69 = Index Array(array=w94, index=w80) -> (element=w90:cluster{dbl[], "Best Polynomial Fit":dbl[]})
              n70 = Reshape Array(w107, w101) -> (→"ellipticity fitting":cluster{dbl[], "best nonlinear fit":dbl[]}[])
              n71 = Reshape Array(w106, w101) -> (→"z signal fitting":cluster{dbl[], "best nonlinear fit":dbl[]}[])
              n72 = Reshape Array(w105, w101) -> (→"x signal fitting":cluster{dbl[], "best nonlinear fit":dbl[]}[])
              n73 = Reshape Array(w104, w101) -> (→"y signal fitting":cluster{dbl[], "best nonlinear fit":dbl[]}[])
              n74 = Bundle(w85, w84) -> (w103:cluster{dbl[], dbl[]})  [unwired: 1 in]
              n75 = Bundle(w112, w116) -> (w111:cluster{dbl[], dbl[]})  [unwired: 1 in]
              n76 = Bundle(w112, w115) -> (w110:cluster{dbl[], dbl[]})  [unwired: 1 in]
              n77 = Bundle(w112, w114) -> (w109:cluster{dbl[], dbl[]})  [unwired: 1 in]
              n78 = Bundle(w112, w113) -> (w108:cluster{dbl[], dbl[]})  [unwired: 1 in]
            }
            "max ellipticity vs power" <- w74
            "var ellipticity vs power" <- w73
            "var x signal vs power" <- w72
            "var y signal vs power" <- w71
            "var z signal vs power" <- w70
            "x DoG" <- w68
            "y DoG" <- w67
            "z DoG" <- w69
          }
          frame #1 {
            # "column name:\n\n0: Cylinder No.\n1: Good? (=1)\n2: K_theta\n3: S_theta\n4: K_e\n5: K_z\n6: S_z\n7: K_zsig\n8: K_x\n9: S_x\n10: K_xsig\n11: K_y\n12: S_y\n13: K_ysig\n14: Max z signal\n15: Max x signal"
            n79 = local read "max ellipticity vs power"() -> (w238:cluster{dbl[], dbl[]}[])
            n80 = for {
              tunnel: w230 -> [w245]
              tunnel: w229 -> [w246] mode=indexing
              tunnel: [w241] -> w228 mode=indexing
              n81 = Index Array(array=w245, index=w246) -> (element=w242:string)
              n82 = Scan Value(string=w242, format string="CylinderNo_%d" ("pattern"), default (0 dbl)=-1) -> (value=w241:i32)  [unwired: 1 out]
            }
            n83 = for {
              tunnel: w231 -> [w275] mode=indexing
              tunnel: [w287] -> w232 mode=indexing
              tunnel: [w286] -> w234 mode=indexing
              tunnel: [w284] -> w235 mode=indexing
              tunnel: [w280] -> w236 mode=indexing
              tunnel: w238 -> [w276] mode=indexing
              tunnel: [w268] -> w226 mode=indexing
              n84 = Unbundle By Name(w275) -> ("z_signal vs trap height slope around eq position, 1/nm"=w299:dbl, "x_signal vs trap height slope around eq position, 1/nm"=w298:dbl, "y_signal vs trap height slope around eq position, 1/nm"=w297:dbl)
              n85 = Unbundle By Name(w275) -> ("height finder result"=w285:cluster{"Y":dbl[], "Y":dbl[]}[], "Z center positon"=w274:dbl, "Z signal Truncated data with redrawn polynomial"=w279:cluster{dbl[], "Best Polynomial Fit":dbl[]}[], "Instrument Calibr.XYZsignal baseline.Zsignal0"=w272:dbl, "X signal Truncated data with redrawn polynomial"=w271:cluster{dbl[], "Best Polynomial Fit":dbl[]}[])
              n86 = Unbundle(w276) -> (w277:dbl[])  [unwired: 1 out]
              n87 = Multiply(x=w277, y=2.0) -> (x*y=w289:dbl[])
              n88 = call-poly <vilib>:"Mean.vi"("X"=w289) -> ("mean"=w288:dbl)  [unwired: 1 out]
              n89 = Index Array(array=w271) -> (element=w270:cluster{dbl[], "Best Polynomial Fit":dbl[]})  [unwired: 1 in]
              n90 = Absolute Value(x=w299) -> (abs(x)=w294:dbl)
              n91 = Absolute Value(x=w298) -> (abs(x)=w295:dbl)
              n92 = Absolute Value(x=w297) -> (abs(x)=w296:dbl)
              n93 = Index Array(array=w285) -> (element #1=w284:cluster{"Y":dbl[], "Y":dbl[]})  [unwired: 2 in, 1 out]
              n94 = Index Array(array=w279, index #2=3 ("index")) -> (element #1=w293:cluster{dbl[], "Best Polynomial Fit":dbl[]})  [unwired: 1 in, 1 out]
              n95 = Unbundle(w270) -> ("Best Polynomial Fit"=w269:dbl[])  [unwired: 1 out]
              n96 = Build Array(w288, w294, w295, w296) -> (w287:dbl[])
              n97 = Unbundle(w293) -> ("Best Polynomial Fit"=w292:dbl[])  [unwired: 1 out]
              n98 = Unbundle(w284) -> ("Y"=w283:dbl[], "Y"=w282:dbl[])
              n99 = Array Max & Min(array=w292) -> (min value=w291:dbl)  [unwired: 3 out]
              n100 = Array Max & Min "max x signal (to calculate max x force)"(array=w269) -> (max value=w268:dbl)  [unwired: 3 out]
              n101 = call "HeightFinder.Fit2.vi"("TrapZ"=w283, "Vsum or Z signal"=w282, "Treat baseline parallel"=TRUE) -> ("bottom position"=w281:dbl)  [unwired: 1 in, 5 out]
              n102 = Subtract "max Delta z signal\n(to calculate max z force)"(x=w272, y=w291) -> (x-y=w286:dbl)
              n103 = Subtract(x=w281, y=w274) -> (x-y=w280:dbl)
            }
            "Height finder data" <- w235
            "distance between trap center and z DoG center" <- w236
            "Array 2" <- w232
            n104 = local read "var ellipticity vs power"() -> (w237:cluster{dbl[], dbl[]}[])
            n105 = local read "var z signal vs power"() -> (w223:cluster{dbl[], dbl[]}[])
            n106 = local read "var x signal vs power"() -> (w222:cluster{dbl[], dbl[]}[])
            n107 = local read "var y signal vs power"() -> (w221:cluster{dbl[], dbl[]}[])
            n108 = Build Array(w237, w223, w222, w221) -> (w239:cluster{dbl[], dbl[]}[][])
            n109 = Transpose 2D Array(2D array=w239) -> (transposed array=w240:cluster{dbl[], dbl[]}[][])
            n110 = for "different cylinders" {
              tunnel: w240 -> [w262] mode=indexing
              tunnel: [w261] -> w225 mode=indexing
              tunnel: [w260] -> w224 mode=indexing
              n111 = for "different signals" {
                tunnel: w262 -> [w267] mode=indexing
                tunnel: [w264] -> w261 mode=indexing
                tunnel: [w263] -> w260 mode=indexing
                n112 = Unbundle(w267) -> (w265:dbl[], w266:dbl[])
                n113 = call <vilib>:"Linear Fit.vi"("Y"=w266, "X"=w265) -> ("slope"=w264:dbl, "intercept"=w263:dbl)  [unwired: 9 in, 3 out]
              }
            }
            "only use slopes" <- w225
            "intercepts that will be ignored" <- w224
            n114 = for {
              tunnel: w225 -> [w255] mode=indexing
              tunnel: w232 -> [w249] mode=indexing
              tunnel: "kT_pNnm" -> [w254]
              tunnel: w234 -> [w251] mode=indexing
              tunnel: w228 -> [w253] mode=indexing
              tunnel: [w250] -> w227 mode=indexing
              tunnel: w226 -> [w247] mode=indexing
              n115 = Square(x=w249) -> (x^2=w258:dbl[])
              n116 = Divide(x=w255, y=w258) -> (x/y=w259:dbl[])
              n117 = Divide "k_theta"(x=w254, y=w259) -> (x/y=w257:dbl[])
              n118 = Divide "K_e"(x=w257, y=w249) -> (x/y=w256:dbl[])
              n119 = Interleave 1D Arrays(w257, w249, w256) -> (w252:dbl[])
              n120 = Build Array (concatenate)(w253, nan ("element"), w252, w251, w247) -> (w250:dbl[])
            }
            "Array" <- w227
          }
          frame #2 {
            # "column name:\n\n0: Cylinder No.\n1: Good? (=1)\n2: K_theta\n3: S_theta\n4: K_e\n5: K_z\n6: S_z\n7: K_zsig\n8: K_x\n9: S_x\n10: K_xsig\n11: K_y\n12: S_y\n13: K_ysig\n14: Max z signal\n15: Max x signal"
            n121 = Array Size(array=w340) -> (size(s)=w341:i32[])
            n122 = Transpose 2D Array(2D array=w340) -> (transposed array=w376:dbl[][])
            "final result" <- w376
            n123 = Index Array(array=w340, index (col) #1=0 ("disabled index (col)"), index (col) #2=4 ("disabled index (col)"), index (col) #3=7 ("index (col)"), index (col) #4=3 ("index (col)"), index (col) #5=6 ("index (col)"), index (col) #6=2 ("index (col)"), index (col) #7=5 ("index (col)"), index (col) #8=9 ("index (col)"), index (col) #9=8 ("index (col)"), index (col) #10=10 ("index (col)")) -> (element #1=w329:dbl[], element #2=w357:dbl[], element #3=w334:dbl[], element #4=w364:dbl[], element #5=w365:dbl[], element #6=w403:dbl[], element #7=w400:dbl[], element #8=w323:dbl[], element #9=w324:dbl[], element #10=w325:dbl[])  [unwired: 10 in]
            n124 = Index Array(array=w341, index=1) -> (element=w343:i32)
            n125 = Decrement(x=w343) -> (x-1=w336:i32)
            n126 = Build Path(base path=w339, name or relative path="result.txt") -> (appended path=w367:path)
            n127 = Decrement(x=w336) -> (x-1=w337:i32)
            n128 = Divide(x=w403, y=2 ("index")) -> (x/y=w405:dbl[])
            n129 = for {
              N -> [w427]
              tunnel: w376 -> [w426] mode=indexing
              tunnel: [w429] -> w425 mode=indexing
              tunnel: [w428] -> w338 mode=indexing
              tunnel: [w427] -> w344
              n130 = call <vilib>:"Std Deviation and Variance.vi"("X"=w426) -> ("mean"=w429:dbl, "standard deviation"=w428:dbl)  [unwired: 1 in, 1 out]
            }
            "mean" <- w425
            "SD" <- w338
            n131 = call-poly <vilib>:"Write To Spreadsheet File.vi"("2D data"=w340, "file path (dialog if empty)"=w367) -> ()  [unwired: 6 in, 1 out]
            n132 = Index Array(array=w340, index (col) #1=w337, index (col) #2=w336) -> (element #1=w335:dbl[], element #2=w333:dbl[])  [unwired: 2 in]
            n133 = Multiply(x=w334, y=w335) -> (x*y=w407:dbl[])
            n134 = Multiply(x=w334, y=w333) -> (x*y=w316:dbl[])
            n135 = Bundle(w329, w357) -> (→"Torque sensitivity":cluster{dbl[], dbl[]})  [unwired: 1 in]
            n136 = Bundle(w329, w334) -> (→"z force sensitivity":cluster{dbl[], dbl[]})  [unwired: 1 in]
            n137 = Bundle(w329, w364) -> (→"Angular sensitivity":cluster{dbl[], dbl[]})  [unwired: 1 in]
            n138 = Bundle(w329, w365) -> (→"z sensitivity":cluster{dbl[], dbl[]})  [unwired: 1 in]
            n139 = Bundle(w329, w403) -> (→"Angular stiffness":cluster{dbl[], dbl[]})  [unwired: 1 in]
            n140 = Bundle(w329, w400) -> (→"z stiffness":cluster{dbl[], dbl[]})  [unwired: 1 in]
            n141 = Bundle(w329, w323) -> (→"x sensitivity":cluster{dbl[], dbl[]})  [unwired: 1 in]
            n142 = Bundle(w329, w324) -> (→"x stiffness":cluster{dbl[], dbl[]})  [unwired: 1 in]
            n143 = Bundle(w329, w325) -> (→"x force sensitivity":cluster{dbl[], dbl[]})  [unwired: 1 in]
            n144 = Bundle(w329, w405) -> (→"Maximum torque":cluster{dbl[], dbl[]})  [unwired: 1 in]
            n145 = Bundle(w329, w407) -> (→"Maximum z force":cluster{dbl[], dbl[]})  [unwired: 1 in]
            n146 = Bundle(w329, w316) -> (→"Maximum x force":cluster{dbl[], dbl[]})  [unwired: 1 in]
            n147 = Square Root(x=w344) -> (sqrt(x)=w317:dbl)
            n148 = call <vilib>:"Std Deviation and Variance.vi"("X"=w407) -> ("mean"=w410:dbl, "standard deviation"=w409:dbl)  [unwired: 1 in, 1 out]
            "max z force, pN/W" <- w410
            "SD of max z force, pN/W" <- w409
            n149 = call <vilib>:"Std Deviation and Variance.vi"("X"=w316) -> ("mean"=w320:dbl, "standard deviation"=w319:dbl)  [unwired: 1 in, 1 out]
            "max x force, pN/W" <- w320
            "SD of max x force, pN/W" <- w319
            n150 = Divide(x=w338, y=w317) -> (x/y=w345:dbl[])
            n151 = Divide(x=w338, y=w425) -> (x/y=w418:dbl[])
            n152 = Divide(x=w409, y=w317) -> (x/y=→"SEM of max z force, pN/W":dbl)
            n153 = Divide(x=w409, y=w410) -> (x/y=→"CV of max z force":dbl)
            n154 = Divide(x=w319, y=w317) -> (x/y=→"SEM of max x force, pN/W":dbl)
            n155 = Divide(x=w319, y=w320) -> (x/y=→"CV of max x force":dbl)
            n156 = Index Array(array=w425, index #1=3 ("index"), index #2=2 ("index"), index #3=6 ("index"), index #4=5 ("index"), index #5=4 ("index"), index #6=7 ("index"), index #7=8 ("index (col)"), index #8=9 ("index (col)")) -> (element #1=→"angular sensitivity, 1/rad":dbl, element #2=→"angular stiffness, pNnm/rad/W":dbl, element #3=→"z sensitivity, 1/nm":dbl, element #4=→"z stiffness, pN/nm/W":dbl, element #5=→"torque sensitivity, pNnm/W":dbl, element #6=→"force sensitivity, pN/W":dbl, element #7=→"x stiffness, pN/nm/W":dbl, element #8=→"z sensitivity, 1/nm 2":dbl)
            n157 = Index Array(array=w345, index #1=3 ("index"), index #2=2 ("index"), index #3=6 ("index"), index #4=5 ("index"), index #5=4 ("index"), index #6=7 ("index"), index #7=8 ("index (col)"), index #8=9 ("index (col)")) -> (element #1=→"SEM of angular sensitivity, 1/rad":dbl, element #2=→"SEM of angular stifness, pNnm/rad/W":dbl, element #3=→"SEM of z sensitivity, 1/nm":dbl, element #4=→"SEM of z stiffness, pN/nm/W":dbl, element #5=→"SEM of torque sensitivity, pNnm/W":dbl, element #6=→"SEM of force sensitivity, pN/W":dbl, element #7=→"SEM of x stiffness, pN/nm/W":dbl, element #8=→"SEM of z sensitivity, 1/nm 2":dbl)
            n158 = Index Array(array=w338, index #1=3 ("index"), index #2=2 ("index"), index #3=6 ("index"), index #4=5 ("index"), index #5=4 ("index"), index #6=7 ("index"), index #7=8 ("index (col)"), index #8=9 ("index (col)")) -> (element #1=→"SD of angular sensitivity, 1/rad":dbl, element #2=→"SD of angular stifness, pNnm/rad/W":dbl, element #3=→"SD of z sensitivity, 1/nm":dbl, element #4=→"SD of z stiffness, pN/nm/W":dbl, element #5=→"SD of torque sensitivity, pNnm/W":dbl, element #6=→"SD of force sensitivity, pN/W":dbl, element #7=→"SD of x stiffness, pN/nm/W":dbl, element #8=→"SD of z sensitivity, 1/nm 2":dbl)
            n159 = Index Array(array=w418, index #1=3 ("index"), index #2=2 ("index"), index #3=6 ("index"), index #4=5 ("index"), index #5=4 ("index"), index #6=7 ("index"), index #7=8 ("index (col)"), index #8=9 ("index (col)")) -> (element #1=→"CV of angular sensitivity":dbl, element #2=→"CV of angular stifness":dbl, element #3=→"CV of z sensitivity":dbl, element #4=→"CV of z stiffness":dbl, element #5=→"CV of torque sensitivity":dbl, element #6=→"CV of force sensitivity":dbl, element #7=→"CV of x stiffness":dbl, element #8=→"CV of z sensitivity 2":dbl)
          }
          frame #3 {
            w442 = "[Comment from " ("search string")
            n160 = local read "angular stiffness, pNnm/rad/W"() -> (w469:dbl)
            n161 = local read "original calibration file"() -> (w436:string)
            n162 = local read "z stiffness, pN/nm/W"() -> (w470:dbl)
            n163 = local read "z sensitivity, 1/nm"() -> (w468:dbl)
            n164 = local read "angular sensitivity, 1/rad"() -> (w466:dbl)
            n165 = local read "mean"() -> (w463:dbl[])
            n166 = Index Array(array=w463, index #1=8, index #2=9, index #3=11, index #4=12) -> (element #1=w458:dbl, element #2=w457:dbl, element #3=w456:dbl, element #4=w455:dbl)
            n167 = Build Array(w458, w457, w456, w455) -> (w454:dbl[])
            n168 = Divide(x=w466, y=2.0) -> (x/y=w465:dbl)
            n169 = Build Array("Kz, pN/nm/W=", "Kang, pNnm/rad/W=", "Sz, 1/nm=", "Max ellipticity, 1=", "Kx, pN/nm/W=", "Sx, 1/nm=", "Ky, pN/nm/W=", "Sy, 1/nm=") -> (w471:string[])
            n170 = local write "pb1"(1.0 ("pb1")) -> ()
            n171 = Build Array (concatenate)(w470, w469, w468, w465, w454) -> (w467:dbl[])
            n172 = for {
              tunnel: w471 -> [w503] mode=indexing
              tunnel: w467 -> [w500] mode=indexing
              shift-right: [w496] -> w447
              shift-left: w436 -> [w506]
              n173 = Search/Split String(string=w506, search string/char (-)=w503) -> (substring before match=w504:string, match + rest of string=w502:string)  [unwired: 1 in, 1 out]
              n174 = Search and Replace String(input string=w502, search string=w503) -> (result string=w501:string)  [unwired: 6 in, 3 out]
              n175 = Scan Value(string=w501, format string="%f", default (0 dbl)=w500) -> (output string=w497:string)  [unwired: 1 out]
              n176 = Format Value(format string="%.6f", value (0)=w500) -> (output string=w498:string)  [unwired: 1 in]
              n177 = Concatenate Strings(w504, w503, w498, w497) -> (w496:string)
            }
            n178 = Search and Replace String(input string=w447, search string=w442, replace string=w442) -> (result string=w448:string, number of replacements=w443:i32, offset past replacement=w449:i32)  [unwired: 5 in, 1 out]
            n179 = Get Date/Time String() -> (date string=w441:string, time string=w439:string)  [unwired: 3 in]
            n180 = case shown="..0" w443 {
              tunnel: w449 -> [_ w484]
              tunnel: w448 -> [w477 w483]
              tunnel: [w478 w481] -> w437
              tunnel: w442 -> [w479 _]
              frame ..0 {
                n181 = call <vilib>:"Trim Whitespace.vi"("string"=w477) -> ("trimmed string"=w476:string)  [unwired: 1 in]
                n182 = Concatenate Strings(w476, "\r\n", w479) -> (w478:string)
              }
              frame 1.. {
                n183 = String Subset(string=w483, offset (0)=0, length (rest)=w484) -> (substring=w481:string)
              }
            }
            n184 = Concatenate Strings(w437, w435, "] " ("string"), w434, "\r\n", w441, " ", w439) -> (w446:string)
            n185 = case shown="No Error" w432 {
              selector: w432 -> [w492 w494]
              tunnel: w446 -> [w486 _]
              tunnel: w431 -> [w493 _]
              tunnel: [w486 "Error! file doesn't exist"] -> w444
              tunnel: [w485 w494] -> w433
              frame No Error {
                n186 = Write to Text File(file (use dialog)=w493, text=w486, error in=w492) -> (refnum out=w488:refnum<file>, error out=w490:errorcluster)  [unwired: 1 in, 1 out]
                n187 = Deny Access(4:w490, 6:T8."deny write-only" ("deny mode (0:deny read/write)"), 7:w488) -> (0:w489:errorcluster, 3:w487:refnum<file>)
                n188 = Close File(refnum=w487, error in=w489) -> (error out=w485:errorcluster)  [unwired: 1 out]
              }
              frame Error {
              }
            }
            "Updated calibration file" <- w444
          }
        }
      }
      event "stop": Value Change; Panel Close {
        n189 = event-data() -> ()  [unwired: 1 in, 1 out]
      }
    }
    "error out" <- w24
  }
  n190 = Unbundle(w14) -> ("status"=w13:bool)  [unwired: 2 out]
  n191 = property on="stop" class="Bool (strict)"("Val(Sgnl)"=w13) -> ()  [unwired: 2 in, 2 out]
